vi "mupGetExprVars.vi"(8 "error in (no error)":errorcluster, 11 "hParser in":u64) -> (0 "error out":errorcluster, 1 "varAddrs":u64[](array[numeric]), 2 "varNames":string[](array[string]), 3 "hParser out":u64, 5 "numVars":i32)   [LabVIEW 2015, in "muParser.lvlib"]
uses:
  muParser.lvlib
  <vilib>/Utility/error.llb/Error Cluster From Error Code.vi
  muparser.dll
  <vilib>/Utility/importsl/GetValueByPointer/GetValueByPointer.xnode
  <vilib>/Utility/importsl/GetValueByPointer/datatype.ctl
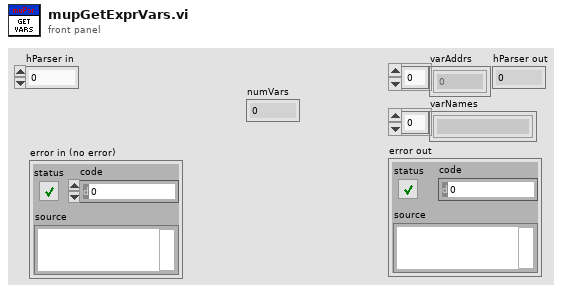
[diagram p1: front panel]
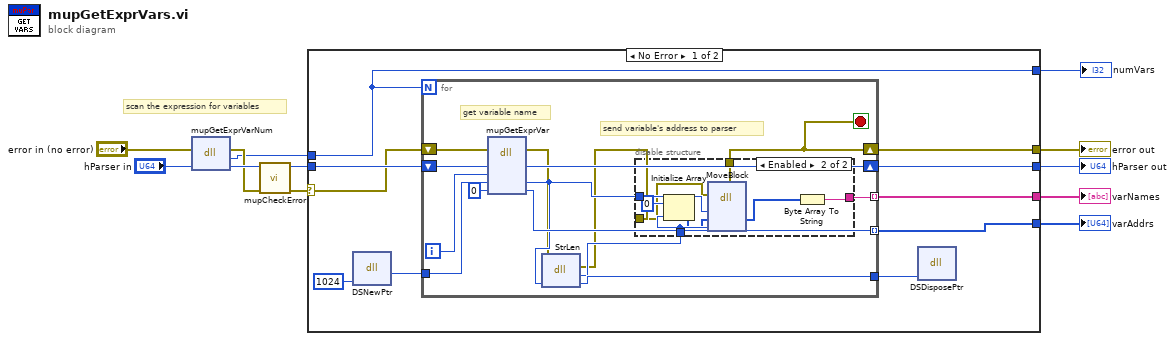
[diagram p0: block diagram]
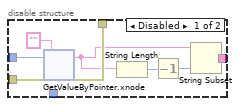
[diagram p2: hidden frame]
diagram:
  # "scan the expression for variables"
  n1 = dll-call lib="C:/Users/porter/Desktop/Projects/muParser/muparser.dll" fn="mupGetExprVarNum"(error in="error in (no error)", "hParser"="hParser in") -> (error out=w11:errorcluster, "return type"=w9:i32, "hParser"=w12:u64)  [unwired: 2 in, 1 out]
  n2 = call "mupCheckError.vi"("error in (no error)"=w11, "hParser in"=w12) -> ("error out"=w2:errorcluster, "hParser out"=w8:u64)  [unwired: 8 in]
  n3 = case shown="No Error" w2 {
    selector: w2 -> [w14 w66]
    tunnel: w9 -> [w13 _]
    tunnel: w8 -> [w20 w65]
    tunnel: [w19 _] -> w7
    tunnel: [w18 _] -> w6
    tunnel: [w17 w66] -> w5
    tunnel: [w15 w65] -> w4
    tunnel: [w13 _] -> w1
    frame No Error {
      n4 = dll-call lib="LabVIEW" fn="DSNewPtr"("size"=1024) -> ("return type"=w21:u64)  [unwired: 4 in, 2 out]
      n5 = for {
        N: w13 -> [_]
        shift-right: [w29] -> w17
        shift-left: w14 -> [w33]
        shift-right: [w31] -> w15
        shift-left: w20 -> [w36]
        tunnel: w21 -> [w34]
        tunnel: [w28] -> w18 mode=indexing
        tunnel: [w30] -> w19 mode=indexing
        tunnel: [w26] -> w16
        i -> [w32]
        stop <- w29 stop-if-true
        # "send variable's address to parser"
        # "get variable name"
        n6 = dll-call lib="C:/Users/porter/Desktop/Projects/muParser/muparser.dll" fn="mupGetExprVar"(error in=w33, "hParser"=w36, "varNum"=w32, "varName"=w34, "varAddr"=u64 0) -> (error out=w24:errorcluster, "hParser"=w31:u64, "varName"=w27:u64, "varAddr"=w30:u64)  [unwired: 4 in, 1 out]
        n7 = dll-call lib="LabVIEW" fn="StrLen"(error in=w24, "pointer"=w27) -> (error out=w23:errorcluster, "return type"=w25:i32, "pointer"=w26:u64)  [unwired: 2 in, 1 out]
        n8 = disable-structure shown="Enabled" {
          disable-tunnel: [w44 w57] -> w29
          disable-tunnel: w23 -> [w43 w58]
          disable-tunnel: w27 -> [w42 w64]
          disable-tunnel: [w37 w60] -> w28
          disable-tunnel: w25 -> [_ w62]
          frame Disabled {
            n9 = xnode "GetValueByPointer.xnode"("Pointer"=w42, "InputType"="", "ErrorIn"=w43) -> ("Output"=w38:string, "ErrorOut"=w44:errorcluster)  [unwired: 1 in]
            n10 = String Length(string=w38) -> (length=w40:i32)
            n11 = Decrement(x=w40) -> (x-1=w39:i32)
            n12 = String Subset(string=w38, length (rest)=w39) -> (substring=w37:string)  [unwired: 1 in]
          }
          frame Enabled {
            n13 = Initialize Array(u8 0 ("Numeric"), w62) -> (w61:u8[])
            n14 = dll-call lib="LabVIEW" fn="MoveBlock"(error in=w58, "ps"=w64, "pd"=w61, "size"=w62) -> (error out=w57:errorcluster, "pd"=w59:u8[])  [unwired: 5 in, 1 out]
            n15 = Byte Array To String(unsigned byte array=w59) -> (string=w60:string)
          }
        }
      }
      n16 = dll-call lib="LabVIEW" fn="DSDisposePtr"("ptr"=w16) -> ()  [unwired: 5 in, 2 out]
    }
    frame Error {
    }
  }
  "varAddrs" <- w7
  "varNames" <- w6
  "error out" <- w5
  "hParser out" <- w4
  "numVars" <- w1
